vi "csv-to-y-x-matrices.vi"(8 "error in (no error)":errorcluster, 11 "Path":path) -> (0 "error out":errorcluster, 1 "X":dbl[][](array[numeric]), 2 "Y":dbl[](array[numeric]), 3 "Title row":string[](array[string]))   [LabVIEW 2023]
uses:
  <vilib>/Utility/file.llb/Read Delimited Spreadsheet (string).vi
  <vilib>/Utility/file.llb/Read Delimited Spreadsheet (DBL).vi
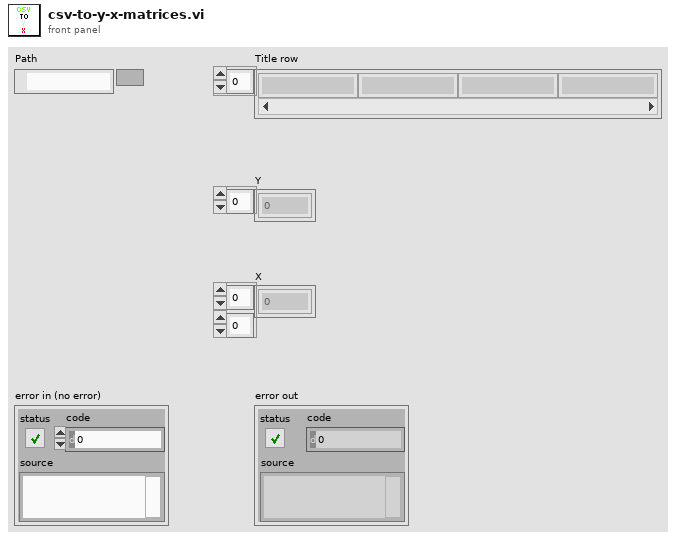
[diagram p1: front panel]
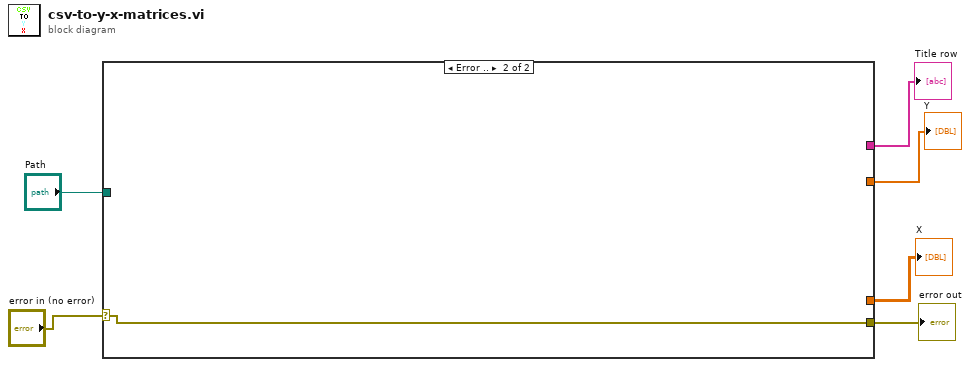
[diagram p0: block diagram]
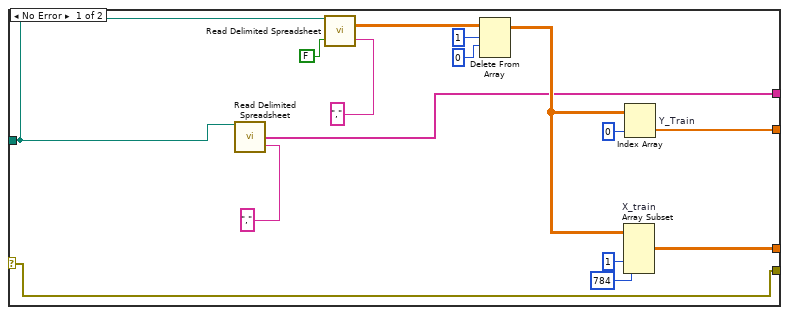
[diagram p2: hidden frame]
diagram:
  n1 = case shown="Error .." "error in (no error)" {
    selector: "error in (no error)" -> [w7 w22]
    tunnel: [w7 w22] -> w2
    tunnel: "Path" -> [w11 _]
    tunnel: [w10 _] -> w4
    tunnel: [w9 _] -> w5
    tunnel: [w8 _] -> w6
    frame No Error {
      n2 = call-poly <vilib>:"Read Delimited Spreadsheet.vi"("file path (dialog if empty)"=w11, "delimiter (\\t)"="," ("delimiter (\\t)")) -> ("first row"=w8:string[])  [unwired: 8 in, 5 out]
      n3 = call-poly <vilib>:"Read Delimited Spreadsheet.vi"("file path (dialog if empty)"=w11, "transpose? (F)"=FALSE, "delimiter (\\t)"="," ("delimiter (\\t)")) -> ("all rows"=w20:dbl[][])  [unwired: 7 in, 5 out]
      n4 = Delete From Array(array=w20, length=1, index (row)=0) -> (array with subset deleted=w21:dbl[][])  [unwired: 1 in, 1 out]
      n5 = Array Subset "X_train"(array=w21, index (col)=1 ("index"), length (col)=784 ("length")) -> (w9:dbl[][])  [unwired: 2 in]
      n6 = Index Array "Y_Train"(array=w21, index (col)=0 ("disabled index (col)")) -> (element=w10:dbl[])  [unwired: 1 in]
    }
    frame Error {
    }
  }
  "error out" <- w2
  "Y" <- w4
  "X" <- w5
  "Title row" <- w6
